vi "Stop Tasks.vi"(8 "error in (no error)":errorcluster, 11 "Series Actor in":refnum<class "Series Actor.lvclass">) -> (0 "error out":errorcluster, 3 "Series Actor out":refnum<class "Series Actor.lvclass">)   [LabVIEW 2023, in "Series Actor.lvlib" / "Series Actor.lvclass"]
uses:
  Series Actor.lvclass
  Series Actor.lvclass/Series Actor.ctl
  Series Base/Series Base.lvclass/Series Base.ctl
  Task/Task Base/Task Base.lvclass/Task Base.ctl
  Series Base/Series Base.lvclass
  Task/Task Base/Task Base.lvclass
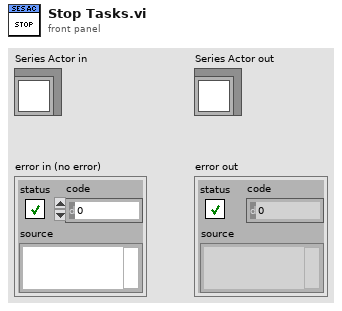
[diagram p1: front panel]
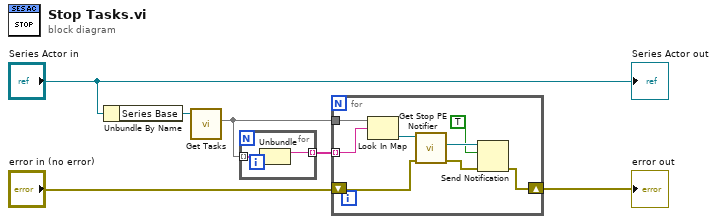
[diagram p0: block diagram]
diagram:
  n1 = Unbundle By Name("Series Actor in") -> ("Series Base"=w5:refnum<class "Series Base.lvclass">)
  n2 = call "Get Tasks.vi"("HAL GOOP4:Series Base in"=w5) -> ("Tasks"=w4:map{string, refnum<class "Task Base.lvclass">})  [unwired: 8 in, 2 out]
  n3 = for {
    tunnel: w4 -> [w8] mode=indexing
    tunnel: [w7] -> w3 mode=indexing
    n4 = Unbundle(w8) -> (w7:string)  [unwired: 1 out]
  }
  n5 = for {
    tunnel: w3 -> [w15] mode=indexing
    tunnel: w4 -> [w16]
    shift-right: [w9] -> w1
    shift-left: "error in (no error)" -> [w13]
    n6 = Look In Map(map=w16, key=w15) -> (value=w14:refnum<class "Task Base.lvclass">)  [unwired: 1 in, 1 out]
    n7 = call "Get Stop PE Notifier.vi"("error in (no error)"=w13, "Task Base in"=w14) -> ("error out"=w10:errorcluster, "Stop PE"=w12:refnum<notifier>)  [unwired: 7 in, 1 out]
    n8 = Send Notification(notification=TRUE, notifier=w12, error in (no error)=w10) -> (error out=w9:errorcluster)  [unwired: 1 out]
  }
  "error out" <- w1
  "Series Actor out" <- "Series Actor in"
